vi "1D_PositionToScalars.vi"(10 "Move to":i32[](array[numeric]), 11 "Move from":i32[](array[numeric])) -> (0 "Column to":i32, 1 "Row to":i32, 2 "Column from":i32, 3 "Row from":i32)   [LabVIEW 2019]
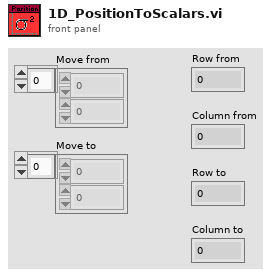
[diagram p1: front panel]
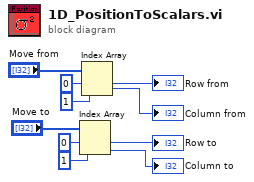
[diagram p0: block diagram]
diagram:
  n1 = Index Array(array="Move to", index #1=0 ("index"), index #2=1 ("index")) -> (element #1=→"Row to":i32, element #2=→"Column to":i32)
  n2 = Index Array(array="Move from", index #1=0 ("index"), index #2=1 ("index")) -> (element #1=→"Row from":i32, element #2=→"Column from":i32)
